vi "ERIO RT Bundle Message.vi"(5 "Position Threshold High":i16, 7 "Position Threshold Low":i16, 8 "State":string, 9 "Previous Position":i16, 10 "Amplitude":dbl format="%#_3g", 11 "Current Position":i16) -> (0 "Output to queue":T1, 1 "Output Position":i16, 3 "Transition Action":T2)   [LabVIEW 2017]
doc: "This VI checks if the current encoder position has passed the threshold for the current stage, and if so will set the Transition Boolean indicator to true. It also bundles position, amplitude, and the stage number string to add to the queue. The consumer loop will then take this information and write the LCD text accordingly.\n\nORIGINAL CODE: \nBy: National Instruments\n NI LabVIEW RIO Evaluation Kit\n Code example \"5- Startup Application\"\n www.ni.com/embeddedsystems\n\nUPDATED CODE: Adds NI SystemLink and NI AWS LabVIEW Tookit functionality for demonstration. \nBy: James Tillett\n Endeavor Engineering Inc.\n www.endeavoreng.com"
uses:
  Controls/ERIO Stage Transition.ctl
  Controls/ERIO Queue Data.ctl
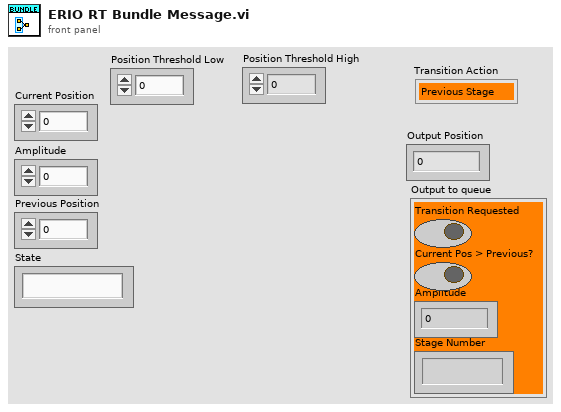
[diagram p1: front panel]
types:
  T1 = typedef "ERIO Queue Data.ctl" = cluster{"Transition Requested":bool, "Current Pos > Previous?":bool, "Amplitude":dbl, "Stage Number":string}
  T2 = typedef "ERIO Stage Transition.ctl" = enum16{"Previous Stage", "Current Stage", "Next Stage"}
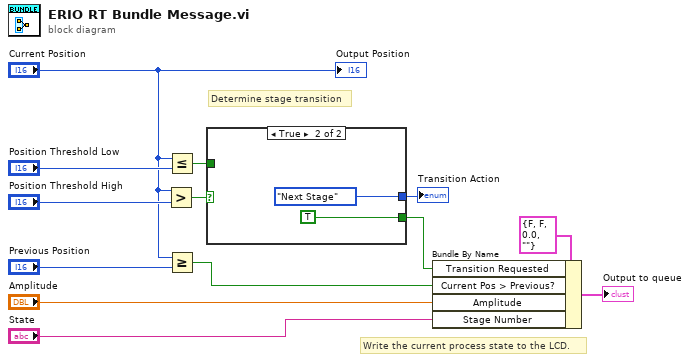
[diagram p0: block diagram]
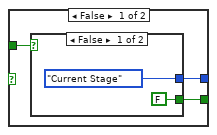
[diagram p2: hidden frame]
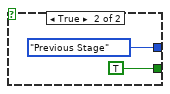
[diagram p3: hidden frame]
diagram:
  # "Determine stage transition"
  # "Write the current process state to the LCD."
  n1 = Greater?(x="Current Position", y="Position Threshold High") -> (0:w6:bool)
  n2 = Less Or Equal?(x="Current Position", y="Position Threshold Low") -> (x <= y?=w3:bool)
  n3 = Greater Or Equal?(x="Current Position", y="Previous Position") -> (x >= y?=w10:bool)
  n4 = case shown="True" w6 {
    tunnel: [w15 ERIO_Stage_Transition."Next Stage" ("Transition Action")] -> w2
    tunnel: w3 -> [w16 _]
    tunnel: [w14 TRUE] -> w1
    frame False {
      n5 = case shown="False" w16 {
        tunnel: [ERIO_Stage_Transition."Current Stage" ("Transition Action") ERIO_Stage_Transition."Previous Stage" ("Transition Action")] -> w15
        tunnel: [FALSE TRUE] -> w14
        frame False {
        }
        frame True {
        }
      }
    }
    frame True {
    }
  }
  "Transition Action" <- w2
  n6 = Bundle By Name(cluster=T1 {"Transition Requested"=FALSE, "Current Pos > Previous?"=FALSE, "Amplitude"=0.0, "Stage Number"=""} ("output to queue"), "Transition Requested"=w1, "Current Pos > Previous?"=w10, "Amplitude"="Amplitude", "Stage Number"="State") -> (→"Output to queue":T1)
  "Output Position" <- "Current Position"
